vi "Pfeiffer_Get_Pressure_Status.vi"(5 "Port":i32(ring) items=["COM 1", "COM 2", "COM 3", "COM 4", "COM 5", "COM 6", "COM 7", "COM 8", "COM 9", "COM 10", "COM 11", "COM 12"], 6 "Error In":bool, 9 "Sensor Nr.:":i32(ring) items=["sensor 1", "sensor 2", "test"]) -> (0 "Pressure":dbl format="%.3e", 1 "Status":i32(ring) items=["data OK", "underrange", "overrange", "sensor error", "sensor off", "no sensor", "ID error"], 4 "Error Out":bool)   [LabVIEW 2010]
doc: "VI runs with Single / Dual Gauge (TPG 252 / 261 / 262)"
panel:
  out "string #2 after point->term":string="03"
  out "string #4 after replace":string
  out "string #3 after substring":string
  out "string #1":string
  # "mbar"
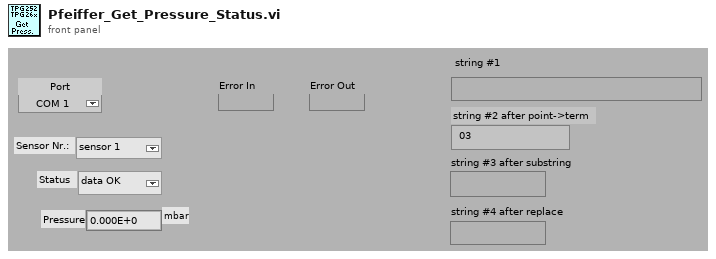
[diagram p1: front panel]
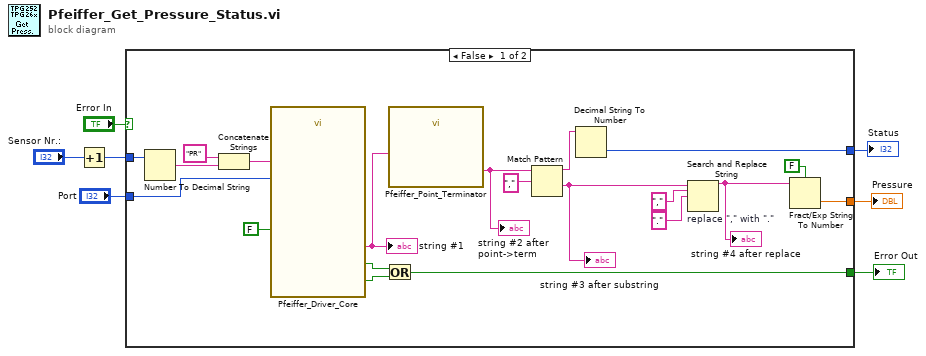
[diagram p0: block diagram]
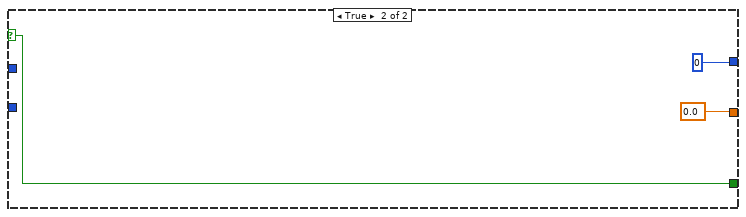
[diagram p2: hidden frame]
diagram:
  n1 = Increment(x="Sensor Nr.:") -> (x+1=w4:i32)
  n2 = case shown="False" "Error In" {
    selector: "Error In" -> [_ w29]
    tunnel: "Port" -> [w27 _]
    tunnel: w4 -> [w26 _]
    tunnel: [w9 0.0] -> w2
    tunnel: [w23 w29] -> w3
    tunnel: [w14 0 ("offset past number")] -> w1
    frame False {
      n3 = Number To Decimal String(number=w26) -> (decimal integer string=w21:string)  [unwired: 1 out]
      n4 = Concatenate Strings("PR", w21) -> (w20:string)
      n5 = call "Pfeiffer_Driver_Core.vi"("Command"=w20, "Write/Read"=FALSE, "Port"=w27) -> ("String Out"=w15:string, "NAK"=w25:bool, "Error"=w24:bool)  [unwired: 2 in, 8 out]
      "string #1" <- w15
      n6 = Or(x=w25, y=w24) -> (x .or. y?=w23:bool)
      n7 = call "Pfeiffer_Point_Terminator.vi"("Eingangstring"=w15) -> ("Ausgangstring"=w19:string)
      "string #2 after point->term" <- w19
      n8 = Match Pattern(string=w19, regular expression=",") -> (before substring=w17:string, after substring=w10:string)  [unwired: 3 out]
      "string #3 after substring" <- w10
      n9 = Decimal String To Number(string=w17) -> (number=w14:i32)  [unwired: 3 out]
      n10 = Search and Replace String "replace \",\" with \".\""(input string=w10, search string="," ("substring (\"\")"), replace string="." ("substring (\"\")")) -> (result string=w11:string)  [unwired: 1 in, 7 out]
      "string #4 after replace" <- w11
      n11 = Fract/Exp String To Number(use system decimal point (T)=FALSE, string=w11) -> (number=w9:dbl)  [unwired: 3 out]
    }
    frame True {
    }
  }
  "Error Out" <- w3
  "Pressure" <- w2
  "Status" <- w1
